vi "CAL-Save Smoothed.vi"(0 "path":path, 5 "Smoothed":dbl[](array[numeric]), 9 "Smooth Params":T1={"Method"=enum."Loess", "MA"={"Iterations"=100, "Length"=3}, "Loess"={"Length"=21, "Type"=enum."Quadratic", "Robust"=TRUE}} {"Loess"."Length" min=1 step=1; "MA"."Length" min=1 step=1; "MA"."Iterations" min=1 step=1}, 11 "error in (no error)":errorcluster) -> (4 "new file path":path, 15 "error out":errorcluster)   [LabVIEW 2020]
uses:
  Type Defs/Cal-Smoothing Parameters.ctl
  epl-vi-lib/Utility VIs/Array Manipulation VIs/Array-Dimensions (2D).vi
  <vilib>/regexp/Match Regular Expression.xnode
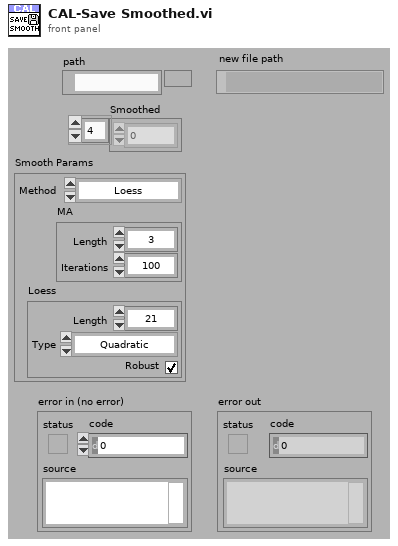
[diagram p1: front panel]
types:
  T1 = typedef "Cal-Smoothing Parameters.ctl" = cluster{"Method":enum16{"None", "Moving average", "Loess"}, "MA":cluster{"Iterations":i32, "Length":i32}, "Loess":cluster{"Length":i32, "Type":enum16{"Linear", "Quadratic"}, "Robust":bool}}
  T2 = enum16{"open", "replace", "create", "open or create", "replace or create", "replace or create with confirmation"}
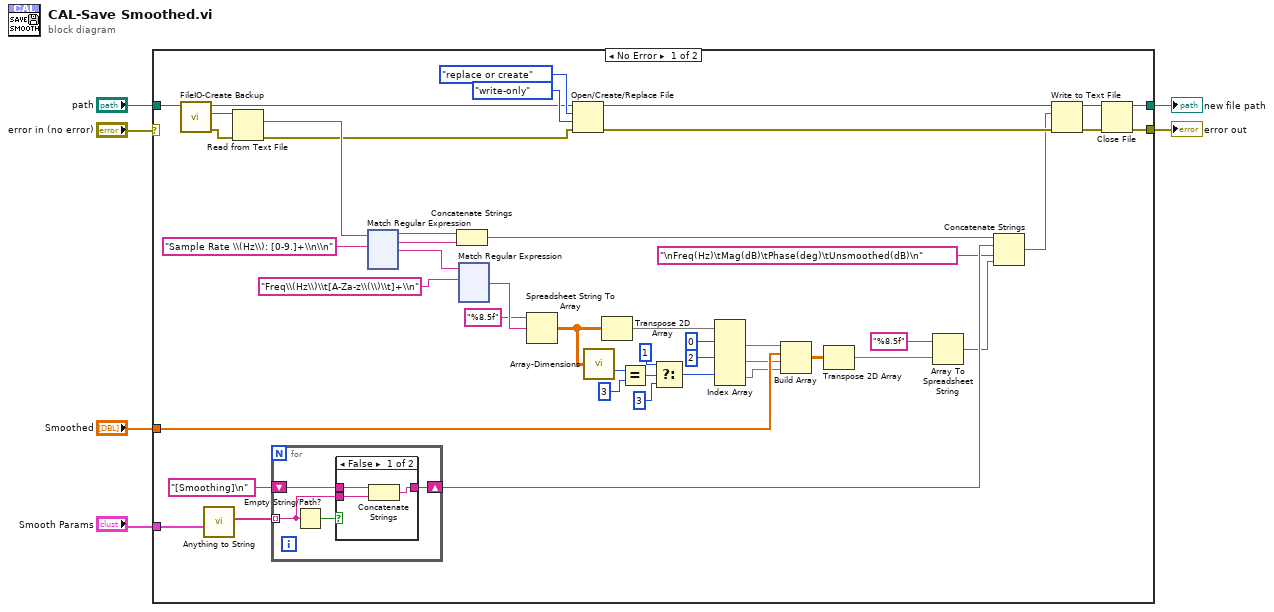
[diagram p0: block diagram]
diagram:
  n1 = case shown="No Error" "error in (no error)" {
    selector: "error in (no error)" -> [_ w283]
    tunnel: [w52 w283] -> w6
    tunnel: [w51 _] -> w4
    tunnel: "path" -> [w44 _]
    tunnel: "Smooth Params" -> [w41 _]
    tunnel: "Smoothed" -> [w23 _]
    frame No Error {
      n2 = call "FileIO-Create Backup.vi"("Path"=w44) -> ("error out"=w47:errorcluster, "Backup Path"=w13:path, "Path (thru)"=w48:path)  [unwired: 7 in, 1 out]
      n3 = call "Anything to String.vi"("Anything"=w41) -> ("Strings[]"=w40:string[])  [unwired: 8 in, 2 out]
      n4 = Read from Text File(file (use dialog)=w13, error in=w47) -> (text=w46:string, error out=w8:errorcluster)  [unwired: 2 in, 2 out]
      n5 = for {
        tunnel: w40 -> [w165] mode=indexing
        shift-right: [w166] -> w11
        shift-left: "[Smoothing]\n" -> [w167]
        n6 = Empty String/Path?(string/path=w165) -> (empty?=w164:bool)
        n7 = case shown="False" w164 {
          tunnel: w167 -> [w170 w171]
          tunnel: w165 -> [w169 _]
          tunnel: [w168 w171] -> w166
          frame False {
            n8 = Concatenate Strings(w170, w169) -> (w168:string)
          }
          frame True {
          }
        }
      }
      n9 = xnode "Match Regular Expression"("input string"=w46, "regular expression"="Sample Rate \\(Hz\\): [0-9.]+\\n\\n") -> ("before match"=w43:string, "whole match"=w42:string, "after match"=w38:string)  [unwired: 4 in, 2 out]
      n10 = Concatenate Strings(w43, w42) -> (w12:string)
      n11 = xnode "Match Regular Expression"("input string"=w38, "regular expression"="Freq\\(Hz\\)\\t[A-Za-z\\(\\)\\t]+\\n") -> ("after match"=w36:string)  [unwired: 4 in, 4 out]
      n12 = Spreadsheet String To Array(format string="%8.5f" ("format (%.3f)"), spreadsheet string=w36) -> (array=w34:dbl[][])  [unwired: 2 in]
      n13 = Open/Create/Replace File(file path (use dialog)=w48, error in=w8, operation (0:open)=T2."replace or create", access (0:read/write)=enum16{"read/write", "read-only", "write-only"}."write-only") -> (refnum out=w15:refnum<file>, error out=w14:errorcluster)  [unwired: 2 in, 1 out]
      n14 = call-poly "Array-Dimensions.vi"("2D Array"=w34) -> ("# columns"=w33:i32)  [unwired: 13 in, 1 out]
      n15 = Transpose 2D Array(2D array=w34) -> (transposed array=w28:dbl[][])
      n16 = Equal?(x=w33, y=3) -> (x = y?=w31:bool)
      n17 = Select(t=1 ("index (col)"), s=w31, f=3 ("index (col)")) -> (s? t:f=w25:i32)
      n18 = Index Array(array=w28, index (row) #1=0 ("disabled index (col)"), index (row) #2=2 ("index (col)"), index (row) #3=w25) -> (element #1=w24:dbl[], element #2=w22:dbl[], element #3=w21:dbl[])  [unwired: 3 in]
      n19 = Build Array(w24, w23, w22, w21) -> (w18:dbl[][])
      n20 = Transpose 2D Array(2D array=w18) -> (transposed array=w19:dbl[][])
      n21 = Array To Spreadsheet String(array=w19, 3:"%8.5f" ("format (%.3f)")) -> (spreadsheet string=w9:string)  [unwired: 1 in]
      n22 = Concatenate Strings(w12, w11, "\nFreq(Hz)\tMag(dB)\tPhase(deg)\tUnsmoothed(dB)\n" ("format string"), w9) -> (w7:string)
      n23 = Write to Text File(file (use dialog)=w15, text=w7, error in=w14) -> (refnum out=w16:refnum<file>, error out=w17:errorcluster)  [unwired: 1 in, 1 out]
      n24 = Close File(refnum=w16, error in=w17) -> (path=w51:path, error out=w52:errorcluster)
    }
    frame Error {
    }
  }
  "error out" <- w6
  "new file path" <- w4
